vi "Open_Instr.vi"(8 "error in (no error)":errorcluster caption="entrée d'erreur (pas d'erreur)", 11 "Class DIO en entrée":refnum<class "Class Instrument Ana.lvclass">) -> (0 "error out":errorcluster caption="sortie d'erreur", 3 "Class DIO en Sortie":refnum<class "Class Instrument Ana.lvclass">)   [LabVIEW 2020, in "Library Instrument & Equipement.lvlib" / "Library Instruments.lvlib" / "Class Instrument Ana.lvclass"]
uses:
  Class Instrument Ana.lvclass
  Class Instrument Ana.lvclass/Class Instrument Ana.ctl
  Instrument (Default)/Class Instrument (Default).lvclass
  Ana/Class Ana (Default)/Class Ana (Default).lvclass
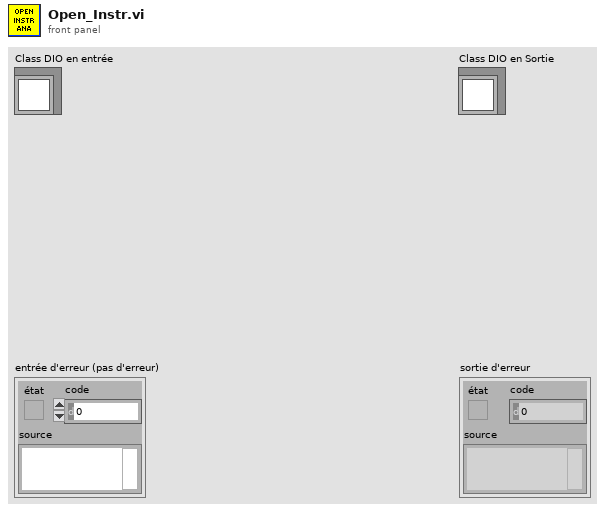
[diagram p1: front panel]
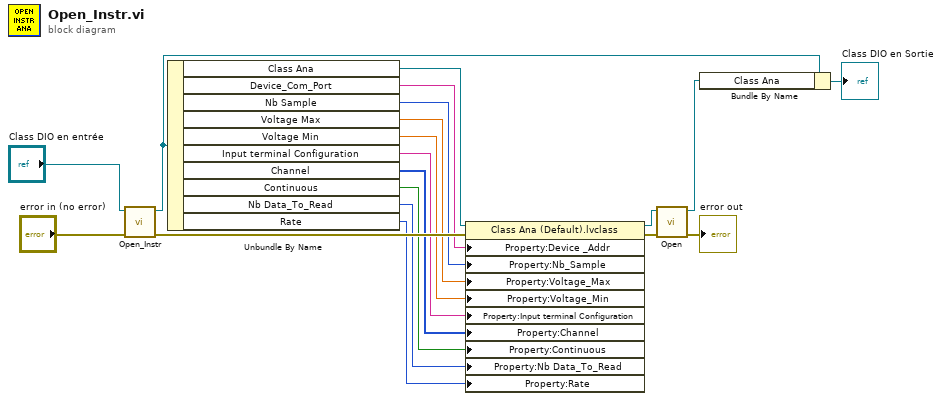
[diagram p0: block diagram]
diagram:
  n1 = call-parent "Open_Instr.vi"("error in (no error)"="error in (no error)", "Class Multimeter (Default) en entrée"="Class DIO en entrée") -> ("error out"=w17:errorcluster, "Class Multimeter (Default) en sortie"=w14:refnum<class "Class Instrument Ana.lvclass">)  [unwired: 8 in]
  n2 = Unbundle By Name(w14) -> ("Class Ana"=w16:refnum<class "Class Ana (Default).lvclass">, "Device_Com_Port"=w15:string, "Nb Sample"=w12:u16, "Voltage Max"=w11:dbl, "Voltage Min"=w10:dbl, "Input terminal Configuration"=w5:string, "Channel"=w2:u8[], "Continuous"=w4:bool, "Nb Data_To_Read"=w3:i16, "Rate"=w1:u16)
  n3 = property class="Class Ana (Default).lvclass"(reference=w16, error in=w17, "Property:Device _Addr"=w15, "Property:Nb_Sample"=w12, "Property:Voltage_Max"=w11, "Property:Voltage_Min"=w10, "Property:Input terminal Configuration"=w5, "Property:Channel"=w2, "Property:Continuous"=w4, "Property:Nb Data_To_Read"=w3, "Property:Rate"=w1) -> (reference out=w9:refnum<class "Class Ana (Default).lvclass">, error out=w8:errorcluster)
  n4 = call-dynamic "Open.vi"("error in (no error)"=w8, "Class DIO (Default) en entrée"=w9) -> ("error out"=→"error out":errorcluster, "Class DIO (Default) en sortie"=w6:refnum<class "Class Ana (Default).lvclass">)  [unwired: 8 in]
  n5 = Bundle By Name(cluster=w14, "Class Ana"=w6) -> (→"Class DIO en Sortie":refnum<class "Class Instrument Ana.lvclass">)
